vi "Configure VI Analyzer.vi"(8 "error in (no error)":errorcluster, 10 "VI Refnum":refnum<vi>[](array[refnum]), 11 "Model in":refnum<class "Model.lvclass">) -> (0 "error out":errorcluster, 3 "Model out":refnum<class "Model.lvclass">)   [LabVIEW 2015, in "Model.lvlib" / "Model.lvclass"]
uses:
  Model.lvclass
  <vilib>/addons/analyzer/NI_VIAnalyzerTKVIs.lvlib
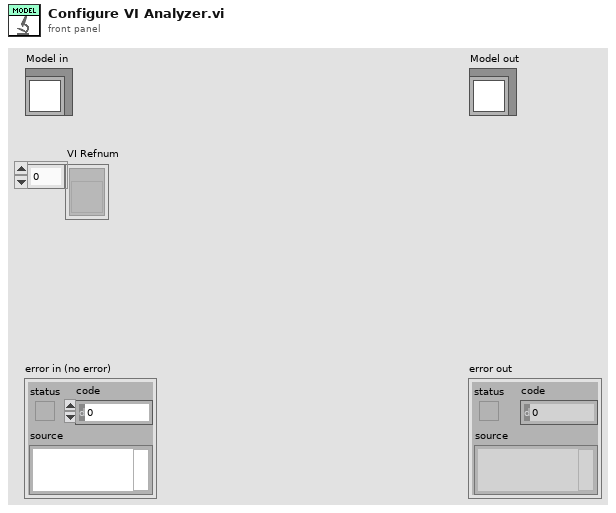
[diagram p1: front panel]
types:
  T1 = typedef "VIAnAPI Ref.ctl" = refnum<k1>
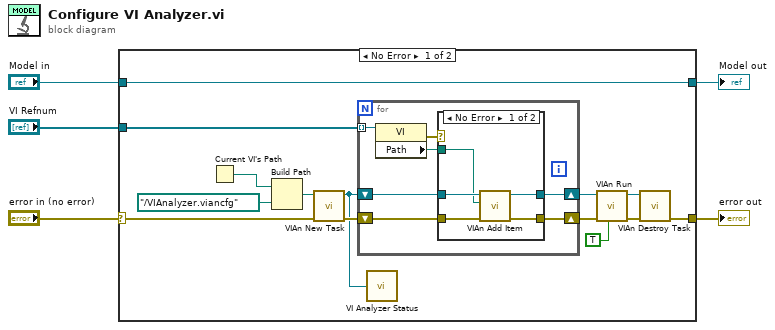
[diagram p0: block diagram]
diagram:
  n1 = case shown="No Error" "error in (no error)" {
    selector: "error in (no error)" -> [w14 w34]
    tunnel: [w13 w35] -> w4
    tunnel: "Model in" -> [w13 w35]
    tunnel: [w9 w34] -> w2
    tunnel: "VI Refnum" -> [w10 _]
    frame No Error {
      n2 = Current VI's Path() -> (path=w12:path)
      n3 = Build Path(base path=w12, name or relative path=path "../VIAnalyzer.viancfg" ("path")) -> (appended path=w19:path)
      n4 = call <vilib>:"VIAn New Task.vi"("error in (no error)"=w14, "Path to Configuration File"=w19) -> ("error out"=w17:errorcluster, "VI Analyzer Task"=w8:T1)  [unwired: 1 in, 7 out]
      n5 = for {
        shift-right: [w24] -> w6
        shift-left: w17 -> [w26]
        shift-right: [w25] -> w15
        shift-left: w8 -> [w23]
        tunnel: w10 -> [w22] mode=indexing
        n6 = property class="VI"(reference=w22) -> (error out=w21:errorcluster, "Path"=w20:path)  [unwired: 1 in, 1 out]
        n7 = case shown="No Error" w21 {
          tunnel: w26 -> [w31 w32]
          tunnel: [w30 w33] -> w25
          tunnel: [w29 w32] -> w24
          tunnel: w23 -> [w28 w33]
          tunnel: w20 -> [w27 _]
          frame No Error {
            n8 = call <vilib>:"VIAn Add Item.vi"("error in (no error)"=w31, "Item to Add"=w27, "VI Analyzer Task in"=w28) -> ("error out"=w29:errorcluster, "VI Analyzer Task out"=w30:T1)  [unwired: 7 out]
          }
          frame Error {
          }
        }
      }
      n9 = call "VI Analyzer Status.vi"("VI Analyzer Task in"=w8) -> ()
      n10 = call <vilib>:"VIAn Run.vi"("Show Results Window?"=TRUE, "error in (no error)"=w6, "VI Analyzer Task in"=w15) -> ("error out"=w7:errorcluster, "VI Analyzer Task out"=w16:T1)  [unwired: 7 out]
      n11 = call <vilib>:"VIAn Destroy Task.vi"("error in (no error)"=w7, "VI Analyzer Task in"=w16) -> ("error out"=w9:errorcluster)  [unwired: 9 out]
    }
    frame Error {
    }
  }
  "error out" <- w2
  "Model out" <- w4
